vi "PDHydra - Breaker AUX & Shunt Trip.vi"(8 "error in (no error)":errorcluster, 10 "Message IN":string) -> (0 "error out":errorcluster, 1 "Result (bool)":bool, 2 "Message OUT":string)   [LabVIEW 2022 SP3]
uses:
  <vilib>/DAQmx/read.llb/DAQmx Read (Digital 1D Bool NChan 1Samp 1Line).vi
  <vilib>/DAQmx/miscellaneous.llb/DAQmx Fill In Error Info.vi
panel:
  in  "bypass":bool
  in  "stop":bool
  out "Expected Breaker AUX state":bool[](array[boolean])
  out "Instructional Message":string
  in  "OK Button":bool
  out "Actual Breaker AUX state":bool[](array[boolean])
  out "Result (color)":u32(colorbox)
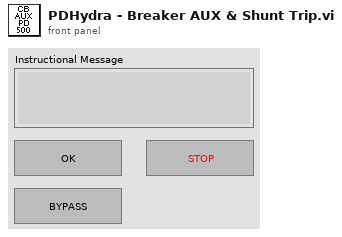
[diagram p1: front panel]
types:
  T1 = cluster{"Expected AUX State":bool[], "Inst. Message":string}[]
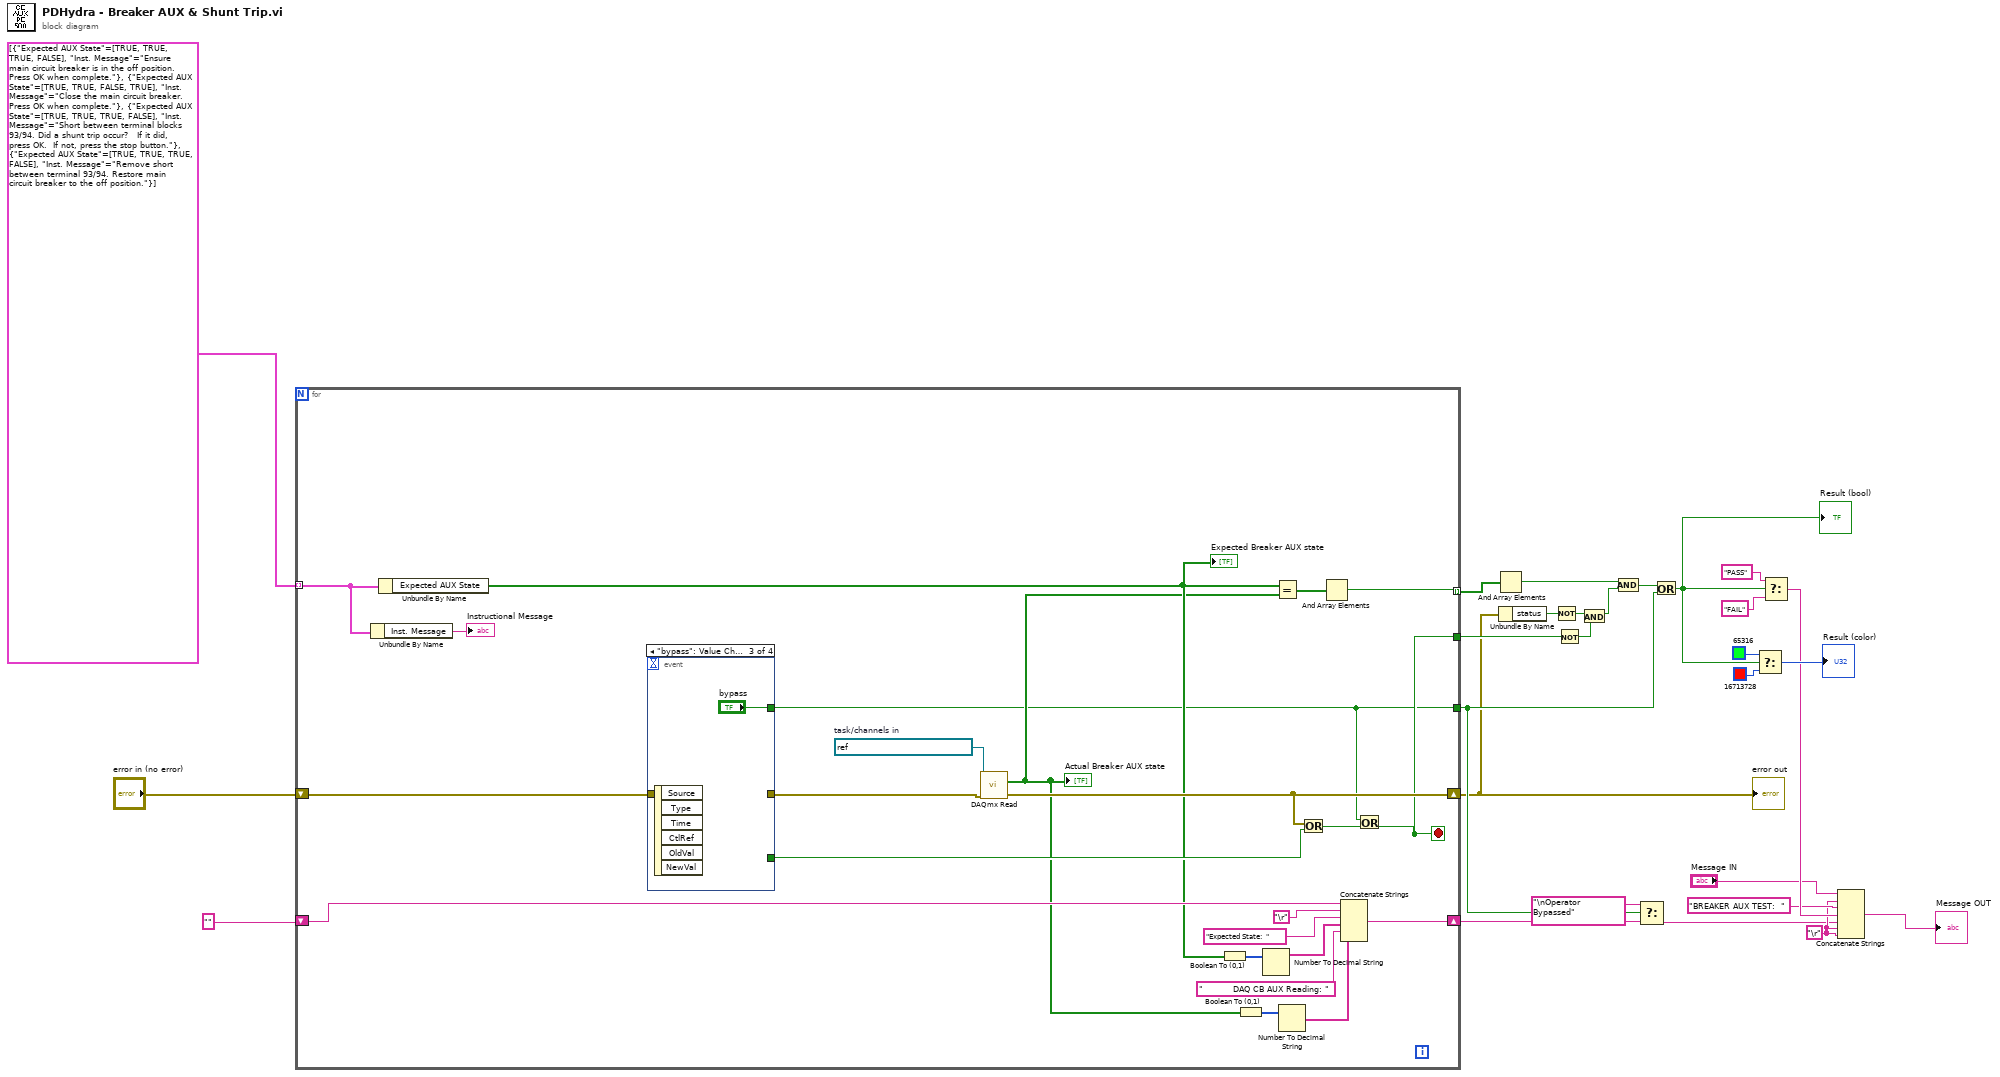
[diagram p0: block diagram]
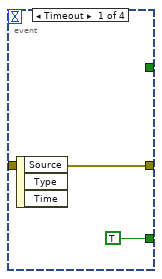
[diagram p2: hidden frame]
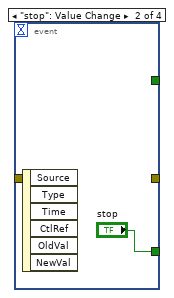
[diagram p3: hidden frame]
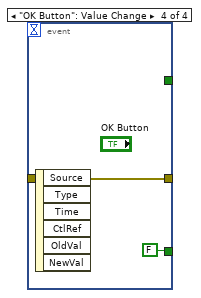
[diagram p4: hidden frame]
diagram:
  w14 = "\r"
  n1 = for {
    shift-right: [w35] -> w1
    shift-left: "error in (no error)" -> [w39]
    tunnel: [w33] -> w27 mode=indexing
    shift-right: [w43] -> w4
    shift-left: "" -> [w42]
    tunnel: T1 [{"Expected AUX State"=[TRUE, TRUE, TRUE, FALSE], "Inst. Message"="Ensure main circuit breaker is in the off position.  Press OK when complete."}, {"Expected AUX State"=[TRUE, TRUE, FALSE, TRUE], "Inst. Message"="Close the main circuit breaker.  Press OK when complete."}, {"Expected AUX State"=[TRUE, TRUE, TRUE, FALSE], "Inst. Message"="Short between terminal blocks 93/94. Did a shunt trip occur?   If it did, press OK.  If not, press the stop button."}, {"Expected AUX State"=[TRUE, TRUE, TRUE, FALSE], "Inst. Message"="Remove short between terminal 93/94. Restore main circuit breaker to the off position."}] -> [w36] mode=indexing
    tunnel: [w29] -> w8
    tunnel: [w28] -> w3
    stop <- w29 stop-if-true
    w40 = refnum<k21> "FTS2_PD500_BreakerAUX"  # task/channels in
    n2 = Unbundle By Name(w36) -> ("Inst. Message"=→"Instructional Message":string)
    n3 = Unbundle By Name(w36) -> ("Expected AUX State"=w31:bool[])
    "Expected Breaker AUX state" <- w31
    n4 = event shown="[2] \"bypass\": Value Change" {
      selector: _ -> [_ _ _ _]
      dyn-events: _ -> [_ _ _ _]
      timeout: _ -> [_ _ _ _]
      tunnel: w39 -> [w52 _ _ w56]
      tunnel: [w52 _ _ w56] -> w38
      tunnel: [TRUE "stop" _ FALSE] -> w34
      tunnel: [_ _ "bypass" _] -> w28
      event Timeout {
        n5 = event-data() -> ()  [unwired: 1 in, 3 out]
      }
      event "stop": Value Change {
        n6 = event-data() -> ()  [unwired: 1 in, 6 out]
      }
      event "bypass": Value Change {
        n7 = event-data() -> ()  [unwired: 1 in, 6 out]
      }
      event "OK Button": Value Change {
        n8 = event-data() -> ()  [unwired: 1 in, 6 out]
      }
    }
    n9 = call-poly <vilib>:"DAQmx Read.vi"("task/channels in"=w40, "error in"=w38) -> ("data"=w30:bool[], "error out"=w35:errorcluster)  [unwired: 11 in, 1 out]
    "Actual Breaker AUX state" <- w30
    n10 = Boolean To (0,1)(Boolean=w31) -> (0, 1=w45:i16[])
    n11 = Boolean To (0,1)(Boolean=w30) -> (0, 1=w44:i16[])
    n12 = Number To Decimal String(number=w45) -> (decimal integer string=w48:string[])  [unwired: 1 in]
    n13 = Equal?(x=w31, y=w30) -> (x = y?=w41:bool[])
    n14 = Number To Decimal String(number=w44) -> (decimal integer string=w50:string[])  [unwired: 1 in]
    n15 = Or(x=w35, y=w34) -> (x .or. y?=w32:bool)
    n16 = And Array Elements(Boolean array=w41) -> (logical AND=w33:bool)
    n17 = Concatenate Strings(w42, "\r", "Expected State:  ", w48, "          DAQ CB AUX Reading: ", w50) -> (w43:string)
    n18 = Or(x=w28, y=w32) -> (x .or. y?=w29:bool)
  }
  "error out" <- w1
  n19 = And Array Elements(Boolean array=w27) -> (logical AND=w19:bool)
  n20 = Unbundle By Name(w1) -> ("status"=w21:bool)
  n21 = Not(x=w21) -> (.not. x?=w20:bool)
  n22 = Not(x=w8) -> (.not. x?=w9:bool)
  n23 = And(x=w20, y=w9) -> (x .and. y?=w10:bool)
  n24 = And(x=w19, y=w10) -> (x .and. y?=w6:bool)
  n25 = Select(t="\nOperator Bypassed", s=w3, f=w4) -> (s? t:f=w5:string)
  n26 = Or(x=w6, y=w3) -> (x .or. y?=w7:bool)
  "Result (bool)" <- w7
  n27 = Select(t=u32 65316 ("Result (color)"), s=w7, f=u32 16713728 ("Result (color)")) -> (s? t:f=→"Result (color)":u32)
  n28 = Select(t="PASS", s=w7, f="FAIL") -> (s? t:f=w17:string)
  n29 = Concatenate Strings("Message IN", w14, "BREAKER AUX TEST:  ", w17, w5, w14, w14) -> (→"Message OUT":string)
